vi "Module Did Stop.vi"(8 "error in (no error)":errorcluster, 10 "Origin":string, 11 "Module ID":i32=-1) -> (0 "error out":errorcluster)   [LabVIEW 2014, in "ConfigurableQMH.lvlib"]
doc: "Send the Module Did Stop event to any VI registered to listen to this module's broadcast events.\n_____\nBased on Delacor QMH Project Template 4.0.0.47."
uses:
  ConfigurableQMH.lvlib
  Stop Argument--cluster.ctl
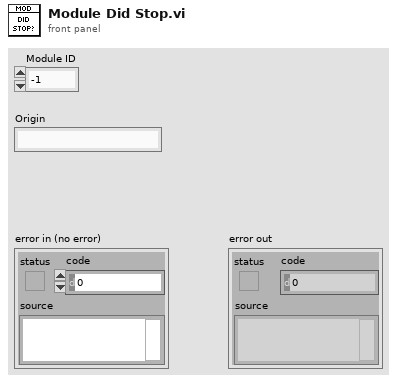
[diagram p1: front panel]
types:
  T1 = typedef "ConfigurableQMH.lvlib/Stop Argument--cluster.ctl" = cluster{"Origin":string, "Module ID":i32, "Exit via Stop Module Req?":bool, "Wait for Module to stop?":bool}
  T2 = typedef "ConfigurableQMH.lvlib/Broadcast Events--cluster.ctl" = cluster{"Module Did Init":refnum<user-event>, "Status Updated":refnum<user-event>, "Error Reported":refnum<user-event>, "Module Did Stop":refnum<user-event>, "Update Module Execution Status":refnum<user-event>, "Module Configuration":refnum<user-event>}
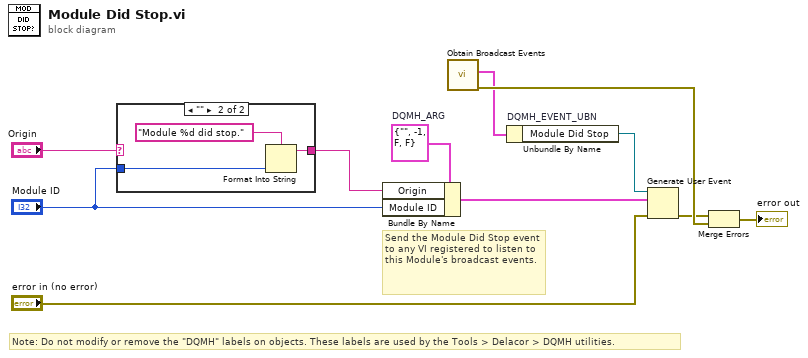
[diagram p0: block diagram]
diagram:
  w4 = T1 {"Origin"="", "Module ID"=-1, "Exit via Stop Module Req?"=FALSE, "Wait for Module to stop?"=FALSE}  # DQMH_ARG
  # "Note: Do not modify or remove the \"DQMH\" labels on objects. These labels are used by the Tools > Delacor > DQMH utilities."
  # "Send the Module Did Stop event to any VI registered to listen to this Module's broadcast events."
  n1 = case shown="\"\"" "Origin" {
    selector: "Origin" -> [w12 _]
    tunnel: "Module ID" -> [_ w15]
    tunnel: [w12 w13] -> w2
    frame Default {
    }
    frame "" {
      n2 = Format Into String(format string="Module %d did stop.", w15) -> (resulting string=w13:string)  [unwired: 2 in, 1 out]
    }
  }
  n3 = Bundle By Name(cluster=w4, "Origin"=w2, "Module ID"="Module ID") -> (w5:T1)
  n4 = call "Obtain Broadcast Events.vi"() -> ("error out"=w9:errorcluster, "ConfigurableQMH Broadcast Events"=w7:T2)  [unwired: 10 in]
  n5 = Unbundle By Name "DQMH_EVENT_UBN"(w7) -> ("Module Did Stop"=w6:refnum<user-event>)
  n6 = Generate User Event(user event=w6, event data cluster=w5, error in="error in (no error)") -> (error out=w8:errorcluster)  [unwired: 1 in, 1 out]
  n7 = Merge Errors(w8, w9) -> (→"error out":errorcluster)
